vi "Add zero to time.vi"(11 "in":string) -> (2 "value 2":string, 3 "value 1":string)   [LabVIEW 2018]
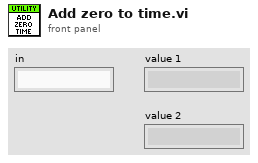
[diagram p1: front panel]
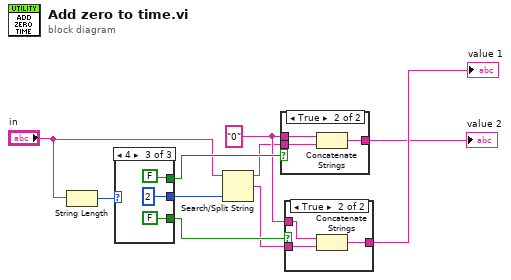
[diagram p0: block diagram]
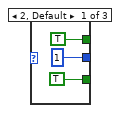
[diagram p4: hidden frame]
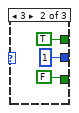
[diagram p5: hidden frame]
diagram:
  w8 = "0" ("string")
  n1 = String Length(string="in") -> (length=w3:i32)
  n2 = case shown="4" w3 {
    tunnel: [1 ("offset (0)") 1 ("offset (0)") 2 ("offset (0)")] -> w1
    tunnel: [TRUE TRUE FALSE] -> w9
    tunnel: [TRUE FALSE FALSE] -> w10
    frame 2, Default {
    }
    frame 3 {
    }
    frame 4 {
    }
  }
  n3 = Search/Split String(string="in", offset (0)=w1) -> (substring before match=w5:string, match + rest of string=w6:string)  [unwired: 1 in, 1 out]
  n4 = case shown="True" w9 {
    tunnel: [w20 w23] -> w4
    tunnel: w5 -> [w20 w22]
    tunnel: w8 -> [_ w21]
    frame False {
    }
    frame True {
      n5 = Concatenate Strings(w21, w22) -> (w23:string)
    }
  }
  "value 2" <- w4
  n6 = case shown="True" w10 {
    tunnel: w6 -> [w24 w27]
    tunnel: [w24 w26] -> w7
    tunnel: w8 -> [_ w25]
    frame False {
    }
    frame True {
      n7 = Concatenate Strings(w25, w27) -> (w26:string)
    }
  }
  "value 1" <- w7
